vi "Configure Filter Averaging.vi"(8 "error in (no error)":errorcluster, 10 "Filter Count (14)":dbl=14.0 min=2.0 max=16.0 step=1.0 format="%#.0p", 11 "VISA resource name":refnum<visa-resource-name>) -> (0 "error out":errorcluster, 3 "VISA resource name out":refnum<visa-resource-name>)   [LabVIEW 2018, in "BK Precision 8600 Series.lvlib"]
doc: "Configures the filter count, which is the number of readings that are acquired and stored in the filter buffer for the averaging calculation for measurement. The larger the filter count, the more filtering that is performed."
uses:
  <instrlib>/BK Precision 8600 Series/BK Precision 8600 Series.lvlib
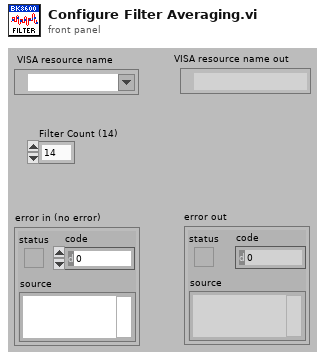
[diagram p1: front panel]
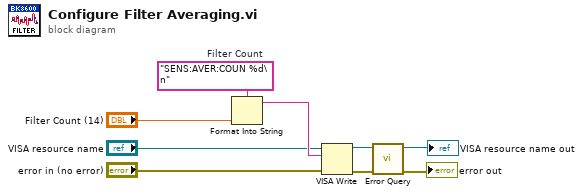
[diagram p0: block diagram]
diagram:
  w6 = "SENS:AVER:COUN %d\n"  # Filter Count
  n1 = Format Into String(format string=w6, "Filter Count (14)") -> (resulting string=w7:string)  [unwired: 2 in, 1 out]
  n2 = VISA Write(VISA resource name="VISA resource name", write buffer=w7, error in (no error)="error in (no error)") -> (VISA resource name out=w5:refnum<visa-resource-name>, error out=w4:errorcluster)  [unwired: 1 out]
  n3 = call <instrlib>:"Error Query.vi"("error in (no error)"=w4, "VISA resource name"=w5) -> ("error out"=→"error out":errorcluster, "VISA resource name out"=→"VISA resource name out":refnum<visa-resource-name>)  [unwired: 6 in, 2 out]
